vi "Write AzPA.vi"(8 "error in (no error)":errorcluster, 10 "AzPA":dbl[unit]=5.817764173314432e-05, 11 "ObjectPA in":refnum<class "ObjectPA.lvclass">) -> (0 "error out":errorcluster, 3 "ObjectPA out":refnum<class "ObjectPA.lvclass">)   [LabVIEW 2014, in "TCSDataDefinitions.lvlib" / "TCSPublicStatus.lvlib" / "PointingPositions.lvlib" / "ObjectPA.lvclass"]
uses:
  ObjectPA.lvclass
  ObjectPA.lvclass/ObjectPA.ctl
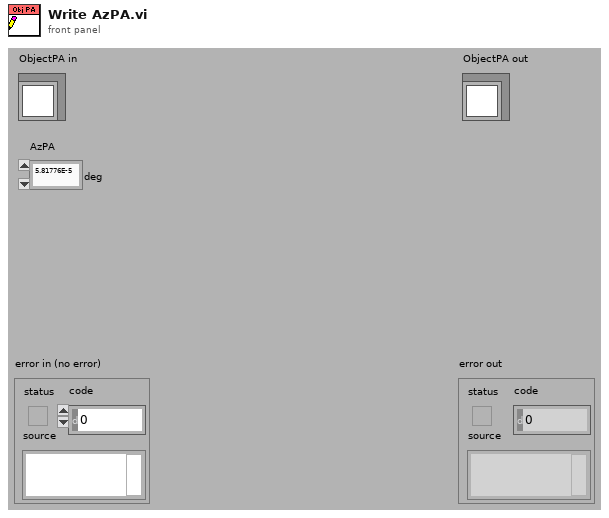
[diagram p1: front panel]
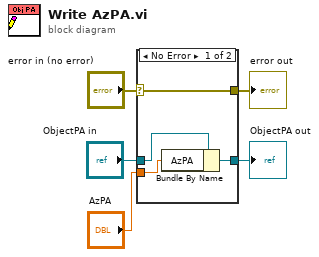
[diagram p0: block diagram]
diagram:
  n1 = case shown="No Error" "error in (no error)" {
    selector: "error in (no error)" -> [w9 w10]
    tunnel: [w9 w10] -> w4
    tunnel: [w7 w11] -> w2
    tunnel: "ObjectPA in" -> [w8 w11]
    tunnel: "AzPA" -> [w6 _]
    frame No Error {
      n2 = Bundle By Name(cluster=w8, "AzPA"=w6) -> (w7:refnum<class "ObjectPA.lvclass">)
    }
    frame Error {
    }
  }
  "error out" <- w4
  "ObjectPA out" <- w2
